vi "DeleteMe.vi"() -> ()   [LabVIEW 2020]
uses:
  controls/Valves Radio.ctl
  <instrlib>/Agilent 34970/Agilent 34970.lvlib
panel:
  in  "Valves Control":T1
  in  "Open/Close (F:Close)":bool=TRUE
  in  "Boolean":bool
  out "error out":errorcluster
  in  "stop":bool
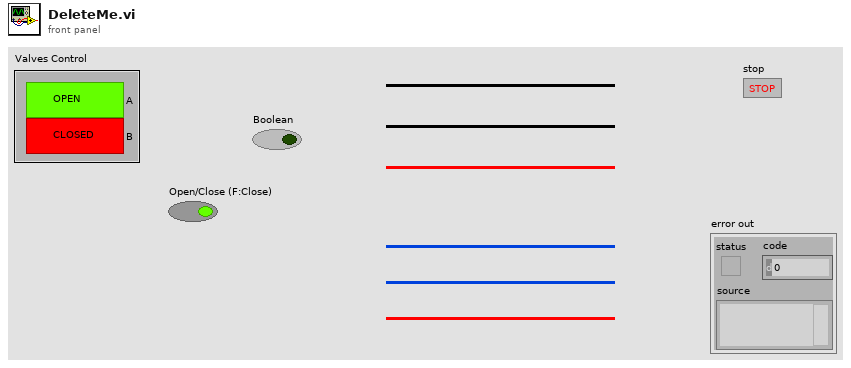
[diagram p1: front panel]
types:
  T1 = typedef "Valves Radio.ctl" = enum32{"A", "B"}
  T2 = cluster{"Timeout Value (10000)":u32, "Baud Rate (57600)":enum16{"1200", "2400", "4800", "9600", "19200", "38400", "57600", "115200"}, "Flow Control (1:XON/XOFF)":enum16{"None", "XON / XOFF", "RTS / CTS", "DTR / DSR"}}
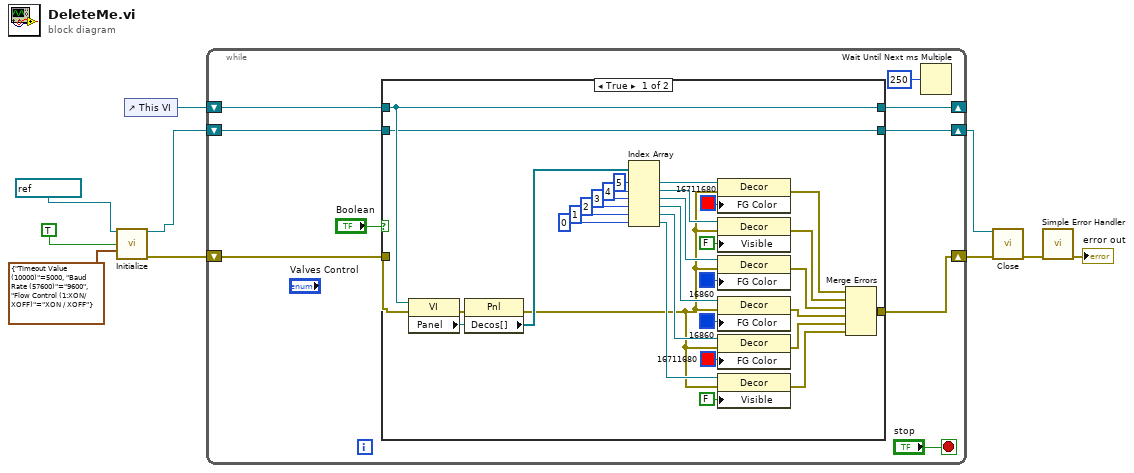
[diagram p0: block diagram]
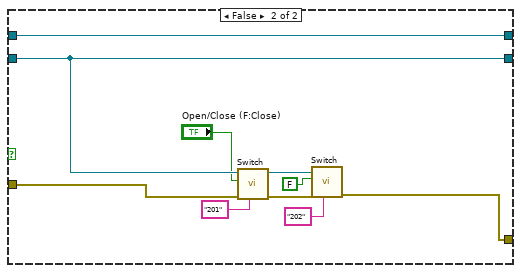
[diagram p2: hidden frame]
diagram:
  n1 = call <instrlib>:"Initialize.vi"("VISA Resource Name"=refnum<visa-resource-name> "34970A" ("VISA resource name"), "Reset (T: Reset)"=TRUE ("Reset"), "Serial Port Configuration"=T2 {"Timeout Value (10000)"=5000, "Baud Rate (57600)"=enum."9600", "Flow Control (1:XON/XOFF)"=enum."XON / XOFF"}) -> ("VISA Resource Name Out"=w6:refnum<visa-resource-name>, "error out"=w5:errorcluster)  [unwired: 11 in]
  n2 = control-ref of="This VI"() -> (w7:refnum<vi>)
  n3 = while {
    shift-right: [w11] -> _
    shift-left: w7 -> [w12]
    shift-right: [w13] -> w3
    shift-left: w6 -> [w14]
    shift-right: [w16] -> w4
    shift-left: w5 -> [w17]
    stop <- "stop" stop-if-true
    n4 = case shown="True" "Boolean" {
      tunnel: w17 -> [w23 w61]
      tunnel: [w22 w56] -> w16
      tunnel: w14 -> [w20 w58]
      tunnel: [w20 w58] -> w13
      tunnel: w12 -> [w21 w59]
      tunnel: [w21 w59] -> w11
      frame True {
        n5 = property class="VI"(reference=w21, error in=w23) -> (error out=w45:errorcluster, "Panel"=w44:refnum<vi>)  [unwired: 1 out]
        n6 = property class="Pnl"(reference=w44, error in=w45) -> (error out=w26:errorcluster, "Decos[]"=w46:refnum<vi>[])  [unwired: 1 out]
        n7 = Index Array(array=w46, index #1=5 ("index"), index #2=4 ("index"), index #3=3 ("index"), index #4=2 ("index"), index #5=1 ("index"), index #6=0 ("index")) -> (element #1=w49:refnum<vi>, element #2=w50:refnum<vi>, element #3=w38:refnum<vi>, element #4=w34:refnum<vi>, element #5=w28:refnum<vi>, element #6=w27:refnum<vi>)
        n8 = property class="Decor"(reference=w49, error in=w26, "FG Color"=u32 16711680) -> (error out=w43:errorcluster)  [unwired: 1 out]
        n9 = property class="Decor"(reference=w50, error in=w26, "Visible"=FALSE) -> (error out=w42:errorcluster)  [unwired: 1 out]
        n10 = property class="Decor"(reference=w38, error in=w26, "FG Color"=u32 16860) -> (error out=w33:errorcluster)  [unwired: 1 out]
        n11 = property class="Decor"(reference=w34, error in=w26, "FG Color"=u32 16860) -> (error out=w32:errorcluster)  [unwired: 1 out]
        n12 = property class="Decor"(reference=w28, error in=w26, "FG Color"=u32 16711680) -> (error out=w25:errorcluster)  [unwired: 1 out]
        n13 = property class="Decor"(reference=w27, error in=w26, "Visible"=FALSE) -> (error out=w24:errorcluster)  [unwired: 1 out]
        n14 = Merge Errors(w43, w42, w33, w32, w25, w24) -> (w22:errorcluster)
      }
      frame False {
        n15 = call <instrlib>:"Switch.vi"("Channel List(empty)"="201", "error in (no error)"=w61, "Open/Close (F:Close)"="Open/Close (F:Close)", "VISA Resource Name"=w58) -> ("error out"=w57:errorcluster, "VISA Resource Name Out"=w53:refnum<visa-resource-name>)  [unwired: 5 in, 1 out]
        n16 = call <instrlib>:"Switch.vi"("Channel List(empty)"="202", "error in (no error)"=w57, "Open/Close (F:Close)"=FALSE, "VISA Resource Name"=w53) -> ("error out"=w56:errorcluster)  [unwired: 5 in, 2 out]
      }
    }
    n17 = Wait Until Next ms Multiple(millisecond multiple=u32 250) -> ()  [unwired: 1 out]
  }
  n18 = call <instrlib>:"Close.vi"("VISA Resource Name"=w3, "error in (no error)"=w4) -> ("error out"=w2:errorcluster)  [unwired: 13 in]
  n19 = call <vilib>:"Simple Error Handler.vi"("error in (no error)"=w2) -> ("error out"=→"error out":errorcluster)  [unwired: 4 in, 4 out]
